vi "Moving Average x8 (SubVI).vi"(0 "Point In":u32, 1 "Boundary Valid? In":bool, 2 "Scan End? In":bool) -> (14 "Point Out":u32, 15 "Boundary Valid? out":bool, 16 "Scan End? Out":bool)   [LabVIEW 2015]
uses:
  Controls (FPGA)/Moving Average.ctl
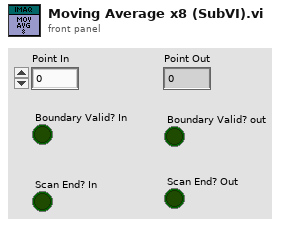
[diagram p1: front panel]
types:
  T1 = typedef "Moving Average.ctl" = enum16{"Enque", "Pass", "Deque"}
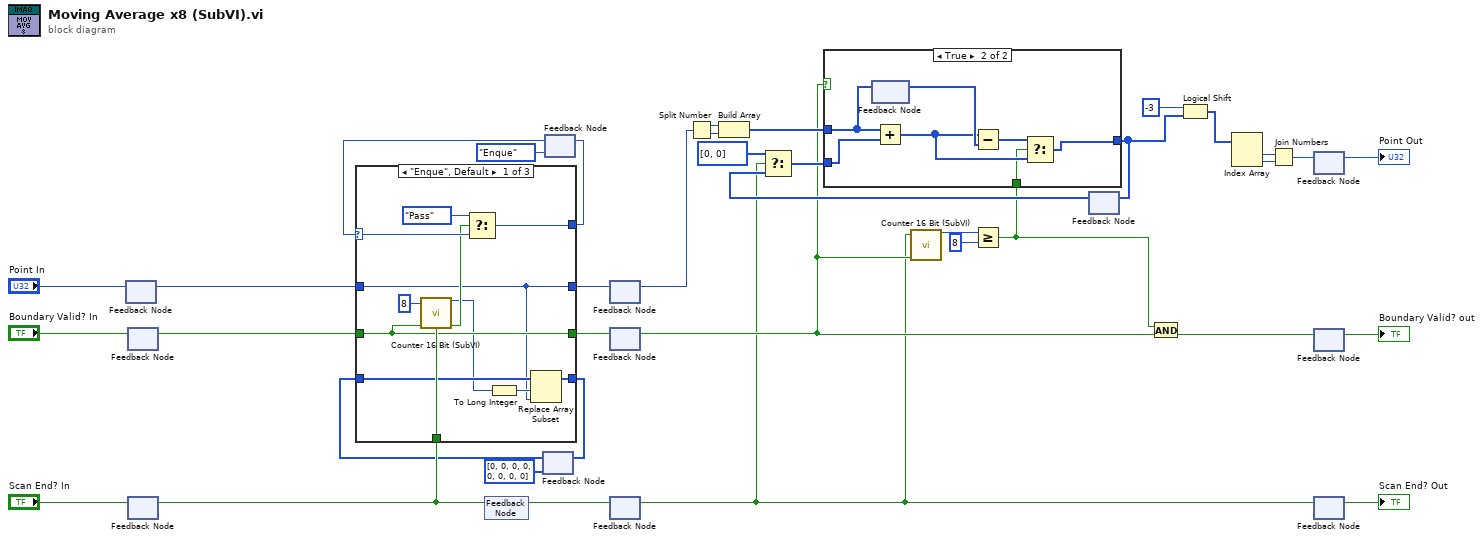
[diagram p0: block diagram]
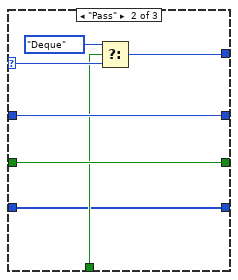
[diagram p2: hidden frame]
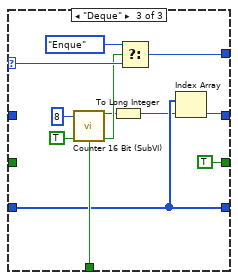
[diagram p3: hidden frame]
diagram:
  n1 = feedback-in #1("Point In") -> ()
  n2 = feedback #1() -> (w1:u32)  [unwired: 1 in]
  n3 = feedback #2() -> (w2:bool)  [unwired: 1 in]
  n4 = feedback-in #2("Boundary Valid? In") -> ()
  n5 = feedback #3() -> (w17:bool)  [unwired: 1 in]
  n6 = feedback-in #3("Scan End? In") -> ()
  n7 = feedback-in #4(w17) -> ()
  n8 = feedback #4() -> (w8:bool)  [unwired: 1 in]
  n9 = feedback #5(u32[] [0, 0, 0, 0, 0, 0, 0, 0]) -> (w10:u32[])
  n10 = feedback #6(Moving_Average."Enque") -> (w19:T1)
  n11 = case shown="\"Enque\", Default" w19 {
    selector: w19 -> [w47 w52 w66]
    tunnel: [w46 w53 w65] -> w20
    tunnel: w2 -> [w43 w56 _]
    tunnel: w17 -> [w44 w51 w63]
    tunnel: w1 -> [w38 w55 _]
    tunnel: [w38 w55 w60] -> w13
    tunnel: [w43 w56 TRUE ("Boundary Valid? In")] -> w16
    tunnel: w10 -> [w42 w50 w62]
    tunnel: [w41 w50 w62] -> w9
    frame "Enque", Default {
      n12 = call "Counter 16 Bit (SubVI).vi"("Max. Count"=u16 8, "RESET"=w44, "Enable"=w43) -> ("Count"=w40:u16, "Count End?"=w45:bool)  [unwired: 10 in, 1 out]
      n13 = Select(t=Moving_Average."Pass", s=w45, f=w47) -> (s? t:f=w46:T1)
      n14 = To Long Integer(number=w40) -> (32bit integer=w39:i32)
      n15 = Replace Array Subset(array=w42, new element=w38, index=w39) -> (w41:u32[])
    }
    frame "Pass" {
      n16 = Select(t=Moving_Average."Deque", s=w51, f=w52) -> (s? t:f=w53:T1)
    }
    frame "Deque" {
      n17 = call "Counter 16 Bit (SubVI).vi"("Max. Count"=u16 8, "RESET"=w63, "Enable"=TRUE) -> ("Count"=w61:u16, "Count End?"=w64:bool)  [unwired: 10 in, 1 out]
      n18 = To Long Integer(number=w61) -> (32bit integer=w58:i32)
      n19 = Select(t=Moving_Average."Enque", s=w64, f=w66) -> (s? t:f=w65:T1)
      n20 = Index Array(array=w62, index=w58) -> (element=w60:u32)
    }
  }
  n21 = feedback-in #5(w9) -> ()
  n22 = feedback-in #6(w20) -> ()
  n23 = feedback-in #7(w13) -> ()
  n24 = feedback #7() -> (w6:u32)  [unwired: 1 in]
  n25 = feedback-in #8(w16) -> ()
  n26 = feedback #8() -> (w7:bool)  [unwired: 1 in]
  n27 = feedback-in #9(w8) -> ()
  n28 = feedback #9() -> (w5:bool)  [unwired: 1 in]
  n29 = Split Number(x=w6) -> (hi(x)=w14:u16, lo(x)=w15:u16)
  n30 = Build Array(w14, w15) -> (w12:u16[])
  n31 = call "Counter 16 Bit (SubVI).vi"("RESET"=w5, "Enable"=w7) -> ("Count"=w31:u16)  [unwired: 11 in, 2 out]
  n32 = Greater Or Equal?(x=w31, y=u16 8) -> (x >= y?=w21:bool)
  n33 = feedback #10() -> (w29:u16[])  [unwired: 1 in]
  n34 = Select(t=u16[] [0, 0], s=w5, f=w29) -> (s? t:f=w24:u16[])
  n35 = case shown="True" w7 {
    tunnel: w12 -> [_ w70]
    tunnel: w21 -> [_ w73]
    tunnel: [w69 w72] -> w28
    tunnel: w24 -> [w69 w71]
    frame False {
    }
    frame True {
      n36 = feedback-in #11(w70) -> ()
      n37 = feedback #11() -> (w76:u16[])  [unwired: 1 in]
      n38 = Add(x=w70, y=w71) -> (x+y=w74:u16[])
      n39 = Subtract(x=w74, y=w76) -> (x-y=w75:u16[])
      n40 = Select(t=w75, s=w73, f=w74) -> (s? t:f=w72:u16[])
    }
  }
  n41 = feedback-in #10(w28) -> ()
  n42 = And(x=w21, y=w7) -> (x .and. y?=w22:bool)
  n43 = Logical Shift(y=i16 -3, x=w28) -> (x << y=w27:u16[])
  n44 = Index Array(array=w27) -> (element #1=w26:u16, element #2=w25:u16)  [unwired: 2 in]
  n45 = Join Numbers(hi=w26, lo=w25) -> ((hi.lo)=w37:u32)
  n46 = feedback-in #12(w37) -> ()
  n47 = feedback #12() -> (→"Point Out":u32)  [unwired: 1 in]
  n48 = feedback-in #13(w22) -> ()
  n49 = feedback #13() -> (→"Boundary Valid? out":bool)  [unwired: 1 in]
  n50 = feedback-in #14(w5) -> ()
  n51 = feedback #14() -> (→"Scan End? Out":bool)  [unwired: 1 in]
